vi "Finalize.vi"(8 "error in":errorcluster, 11 "Tx Execution Unit in":refnum<class "Tx Generic Execution Unit.lvclass">) -> (0 "error out":errorcluster, 3 "Tx Execution Unit out":refnum<class "Tx Generic Execution Unit.lvclass">)   [LabVIEW 2020, in "AIM ARINC 664 Engine.lvlib" / "Implementation.lvlib" / "Tx Generic Execution Unit.lvclass"]
uses:
  Tx Generic Execution Unit.lvclass
  Program Files/National Instruments/LabVIEW 2024/instr.lib/AIM GmbH/_AIM 664/AIM664LV.lvlib
  Program Files/National Instruments/LabVIEW 2024/instr.lib/AIM GmbH/_AIM 664/bsp/Fdx Stop (Tx).vi
  <vilib>/Utility/SystemLogging/NI_SystemLogging.lvlib
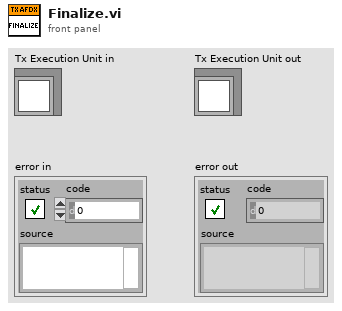
[diagram p1: front panel]
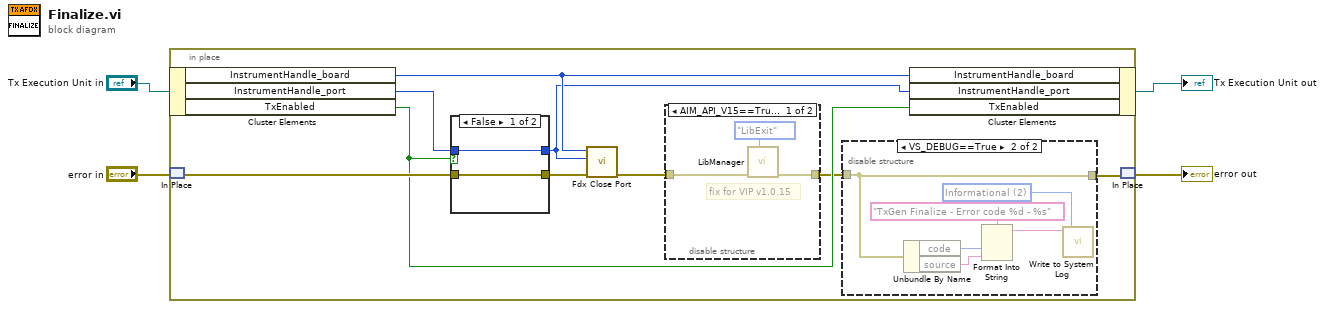
[diagram p0: block diagram]
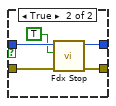
[diagram p4: hidden frame]
diagram:
  n1 = in-place {
    n2 = in-place-cluster #1("Tx Execution Unit in") -> ("InstrumentHandle_board"=w13:u32, "InstrumentHandle_port"=w12:u32, "TxEnabled"=w8:bool)
    n3 = in-place-match #2("error in") -> (w11:errorcluster)
    n4 = case shown="False" w8 {
      tunnel: w12 -> [w26 w31]
      tunnel: w11 -> [w25 w29]
      tunnel: [w25 w28] -> w10
      tunnel: [w26 w27] -> w9
      frame False {
      }
      frame True {
        n5 = call-poly "Fdx Stop.vi"("error in"=w29, "Force Stop?"=TRUE, "InstrumentHandle_port in"=w31) -> ("error out"=w28:errorcluster, "InstrumentHandle_port out"=w27:u32)  [unwired: 7 in]
      }
    }
    n6 = call "Fdx Close Port.vi"("error in"=w10, "InstrumentHandle_port in"=w9, "InstrumentHandle_board in"=w13) -> ("error out"=w7:errorcluster)  [unwired: 7 in, 1 out]
    n7 = disable-structure shown="AIM_API_V15==True" {
      disable-tunnel: w7 -> [w23 w24]
      disable-tunnel: [w22 w24] -> w6
      frame condition #0 {
        # "fix for VIP v1.0.15"
        n8 = call "LibManager.vi"("action"=enum16{"LibInit", "LibExit"}."LibExit", "error in (no error)"=w23) -> ("error out"=w22:errorcluster)  [unwired: 7 in, 2 out]
      }
      frame condition #1 (active) {
      }
    }
    n9 = disable-structure shown="VS_DEBUG==True" {
      disable-tunnel: w6 -> [w14 w15]
      disable-tunnel: [w14 w15] -> w5
      frame condition #0 (active) {
      }
      frame condition #1 {
        w18 = 2 items=["Error", "Warning", "Informational"] ("severity")
        n10 = Unbundle By Name(w15) -> ("code"=w17:i32, "source"=w16:string)
        n11 = Format Into String(format string="TxGen Finalize - Error code %d - %s", w17, w16) -> (resulting string=w19:string)  [unwired: 2 in, 1 out]
        n12 = call <vilib>:"Write to System Log.vi"("severity"=w18, "message"=w19) -> ()  [unwired: 9 in, 1 out]
      }
    }
    n13 = in-place-cluster #1("InstrumentHandle_board"=w13, "InstrumentHandle_port"=w9, "TxEnabled"=w8) -> (→"Tx Execution Unit out":refnum<class "Tx Generic Execution Unit.lvclass">)
    n14 = in-place-match #2(w5) -> (→"error out":errorcluster)
  }
